vi "DisplayName(GetDisplayName3).vi"(0 "XRef":T4, 1 "State In":T3={"Type"=variant(bool FALSE), "Name Type"=enum."String"}) -> (14 "Type Name":T2, 15 "Instance Name":T2, 16 "Fatal Error Out":T1)   [LabVIEW 2014, in "TagDB(dev).lvlib" / "tagDB_value.xnode"]
uses:
  tagDB_value.xnode
  <vilib>/XNodeSupport/XNodeXNodeRef.ctl
  State.ctl
  <vilib>/XNodeSupport/XNodeString.ctl
  <vilib>/XNodeSupport/XNodeErrorCluster.ctl
  <vilib>/XNodeSupport/NI_XNodeSupport.lvlib
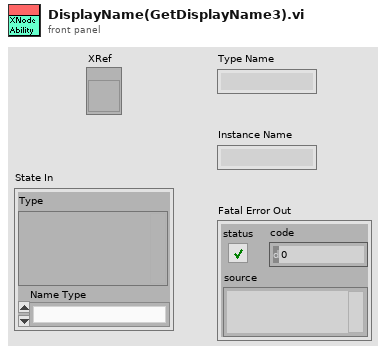
[diagram p1: front panel]
types:
  T1 = typedef "NI_XNodeSupport.lvlib/XNodeErrorCluster.ctl" = errorcluster
  T2 = typedef "NI_XNodeSupport.lvlib/XNodeString.ctl" = string
  T3 = typedef "TagDB(dev).lvlib/tagDB_value.xnode/State.ctl" = cluster{"Type":variant, "Name Type":enum16{"String", "RegPattern"}}
  T4 = typedef "NI_XNodeSupport.lvlib/XNodeXNodeRef.ctl" = refnum<vi>
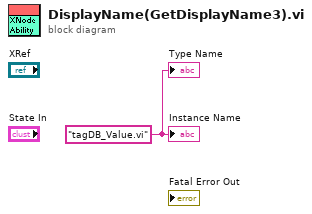
[diagram p0: block diagram]
diagram:
  w1 = T2 "tagDB_Value.vi" ("Instance Name")
  "Type Name" <- w1
  "Instance Name" <- w1
